vi "Line Intersection.vi"(8 "error in (no error)":errorcluster, 9 "Straight Edges 2":T2(array[cluster]), 10 "Straight Edges 1":T2(array[cluster]), 11 "Image in":T1) -> (0 "error out":errorcluster, 1 "Angle":dbl format="%.2f", 2 "Intersection Point":cluster{"X":sgl, "Y":sgl} {"Y" format="%.2f"; "X" format="%.2f"}, 3 "Image Out":T1)   [LabVIEW 2017]
uses:
  <vilib>/vision/Image Controls.llb/IMAQ Image.ctl
  <vilib>/vision/NI_Vision_Development_Module.lvlib
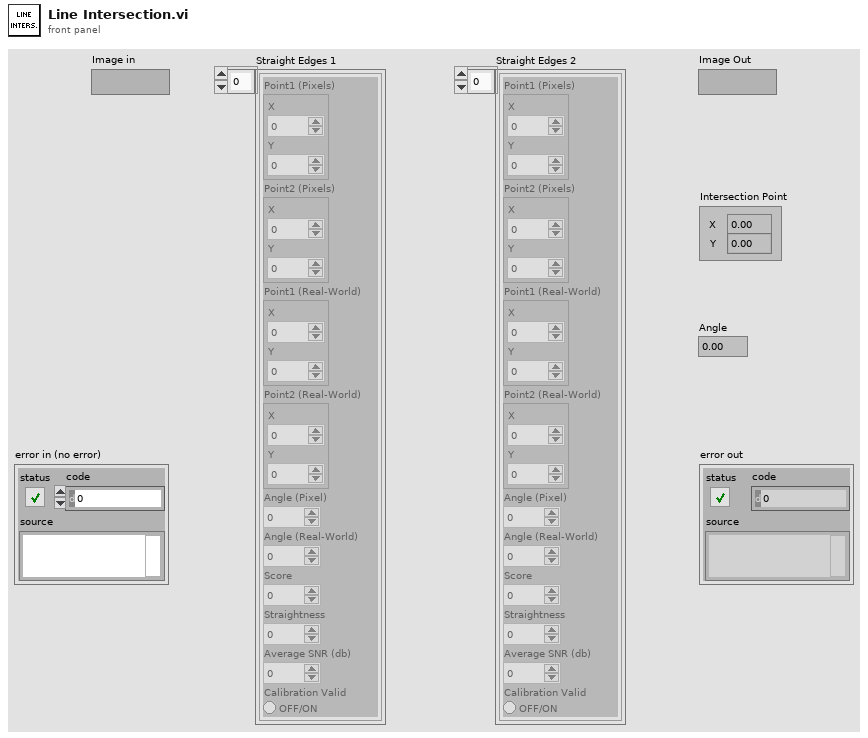
[diagram p1: front panel]
types:
  T1 = typedef "IMAQ Image.ctl" = refnum<image>
  T2 = cluster{"Point1 (Pixels)":cluster{"X":sgl, "Y":sgl}, "Point2 (Pixels)":cluster{"X":sgl, "Y":sgl}, "Point1 (Real-World)":cluster{"X":sgl, "Y":sgl}, "Point2 (Real-World)":cluster{"X":sgl, "Y":sgl}, "Angle (Pixel)":dbl, "Angle (Real-World)":dbl, "Score":dbl, "Straightness":dbl, "Average SNR (db)":dbl, "Calibration Valid":bool}[]
  T3 = cluster{"Point1 (Pixels)":cluster{"X":sgl, "Y":sgl}, "Point2 (Pixels)":cluster{"X":sgl, "Y":sgl}, "Point1 (Real-World)":cluster{"X":sgl, "Y":sgl}, "Point2 (Real-World)":cluster{"X":sgl, "Y":sgl}, "Angle (Pixel)":dbl, "Angle (Real-World)":dbl, "Score":dbl, "Straightness":dbl, "Average SNR (db)":dbl, "Calibration Valid":bool}
  T4 = cluster{"Point1 (Pixels)":cluster{"X":sgl, "Y":sgl}, "Point2 (Pixels)":cluster{"X":sgl, "Y":sgl}}
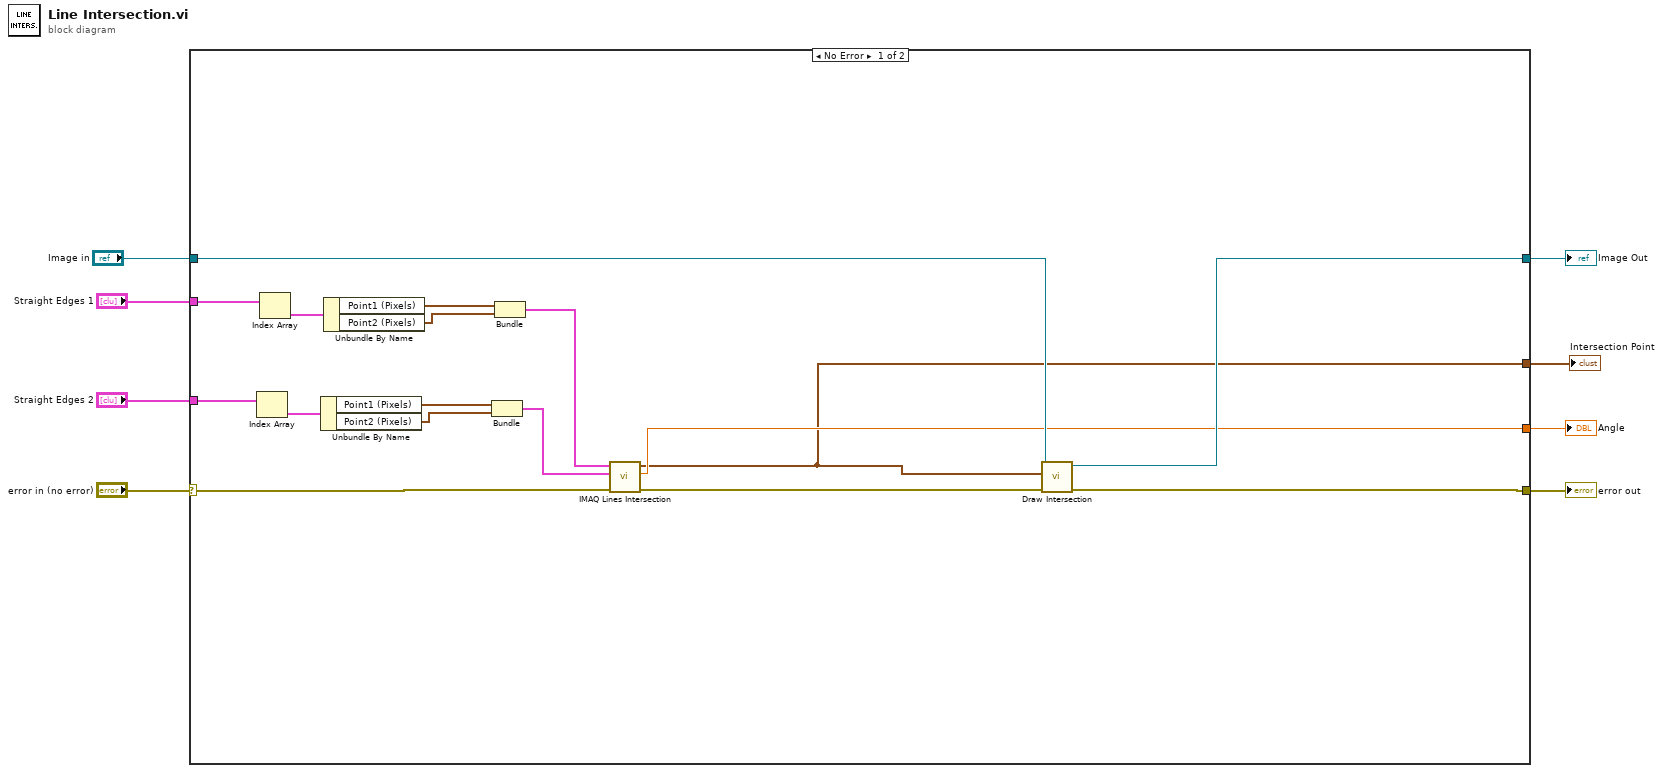
[diagram p0: block diagram]
diagram:
  n1 = case shown="No Error" "error in (no error)" {
    selector: "error in (no error)" -> [w25 w27]
    tunnel: [w11 w27] -> w7
    tunnel: "Straight Edges 1" -> [w24 _]
    tunnel: "Straight Edges 2" -> [w17 _]
    tunnel: [w10 _] -> w4
    tunnel: "Image in" -> [w14 w26]
    tunnel: [w13 w26] -> w2
    tunnel: [w9 _] -> w1
    frame No Error {
      n2 = Index Array(array=w17) -> (element=w20:T3)  [unwired: 1 in]
      n3 = Index Array(array=w24) -> (element=w23:T3)  [unwired: 1 in]
      n4 = Unbundle By Name(w20) -> ("Point1 (Pixels)"=w19:cluster{"X":sgl, "Y":sgl}, "Point2 (Pixels)"=w18:cluster{"X":sgl, "Y":sgl})
      n5 = Unbundle By Name(w23) -> ("Point1 (Pixels)"=w22:cluster{"X":sgl, "Y":sgl}, "Point2 (Pixels)"=w21:cluster{"X":sgl, "Y":sgl})
      n6 = Bundle("Point1 (Pixels)"=w19, "Point2 (Pixels)"=w18) -> (w16:T4)  [unwired: 1 in]
      n7 = Bundle("Point1 (Pixels)"=w22, "Point2 (Pixels)"=w21) -> (w15:T4)  [unwired: 1 in]
      n8 = call "IMAQ Lines Intersection"("error in (no error)"=w25, "Line 2"=w16, "Line 1"=w15) -> ("error out"=w12:errorcluster, "Angle"=w10:dbl, "Intersection Point"=w9:cluster{"X":sgl, "Y":sgl})  [unwired: 6 in]
      n9 = call "Draw Intersection.vi"("error in (no error)"=w12, "Intersection Point"=w9, "Refnum in"=w14) -> ("error out"=w11:errorcluster, "Refnum out"=w13:T1)  [unwired: 7 in]
    }
    frame Error {
    }
  }
  "error out" <- w7
  "Angle" <- w4
  "Image Out" <- w2
  "Intersection Point" <- w1
